vi "VGC Defaults.vi"() -> (3 "Data":T1={"UI References"={"Exit Ref"=refnum, "Save Ref"=refnum, "Export Ref"=refnum, "Acquire Ref"=refnum, "Configure Ref"=refnum, "Graph Ref"=refnum, "Analyze Ref"=refnum, "Status Ref"=refnum, "Snapshot Ref"=refnum, "Start Ref"=refnum}, "Vacuum Graph config"={"Log/Lin"=FALSE, "Show Backing"=FALSE, "Show Chamber"=FALSE}, "VGC50"={"serial settings"={"port"="Inficon_VGC503", "baud rate"=115200}, "device information"={"type"="", "model number"="", "serial number"="", "firmware version"="", "hardware version"=""}, "VGC"=refnum, "Backing SP"={"mode"=2, "thresholds"={"lower"=0.1, "upper"=1.0}, "on"=FALSE}, "Chamber SP"={"mode"=3, "thresholds"={"lower"=1e-05, "upper"=0.0001}, "on"=FALSE}}} {"VGC50"."Chamber SP"."thresholds"."upper" format="%#_5p"; "VGC50"."Chamber SP"."thresholds"."lower" format="%#_5p"; "VGC50"."Chamber SP"."mode" items=["off", "on", "channel 1", "channel 2", "channel 3"]; "VGC50"."Backing SP"."thresholds"."upper" format="%#_5p"; "VGC50"."Backing SP"."thresholds"."lower" format="%#_5p"; "VGC50"."Backing SP"."mode" items=["off", "on", "channel 1", "channel 2", "channel 3"]; "VGC50"."serial settings"."baud rate" items=["9600"=9600, "19200"=19200, "38400"=38400, "57600"=57600, "115200"=115200]})   [LabVIEW 2024]
uses:
  controls/UI References.ctl
  controls/Vac Graph Config.ctl
  Program Files/National Instruments/LabVIEW 2024/instr.lib/PL Inficon VGC/PL Inficon VGC.lvclass
  controls/VGC50.ctl
  controls/VGCData.ctl
panel:
  in  "VGC50":T4={"serial settings"={"port"="Inficon_VGC503", "baud rate"=115200}, "device information"={"type"="", "model number"="", "serial number"="", "firmware version"="", "hardware version"=""}, "VGC"=refnum, "Backing SP"={"mode"=2, "thresholds"={"lower"=0.0001, "upper"=0.005}, "on"=FALSE}, "Chamber SP"={"mode"=3, "thresholds"={"lower"=1e-05, "upper"=0.0001}, "on"=FALSE}} {"Chamber SP"."thresholds"."upper" format="%#_5p"; "Chamber SP"."thresholds"."lower" format="%#_5p"; "Chamber SP"."mode" items=["off", "on", "channel 1", "channel 2", "channel 3"]; "Backing SP"."thresholds"."upper" format="%#_5p"; "Backing SP"."thresholds"."lower" format="%#_5p"; "Backing SP"."mode" items=["off", "on", "channel 1", "channel 2", "channel 3"]; "serial settings"."baud rate" items=["9600"=9600, "19200"=19200, "38400"=38400, "57600"=57600, "115200"=115200]}
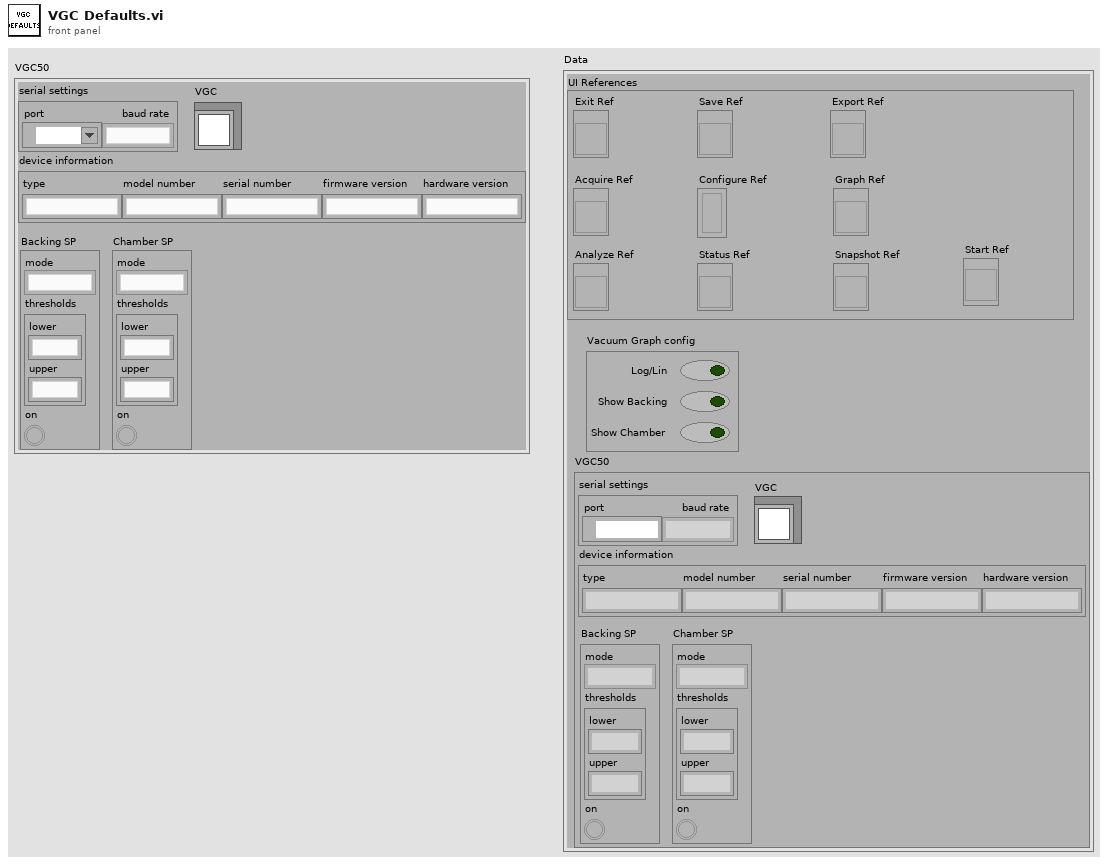
[diagram p1: front panel]
types:
  T1 = typedef "VGCData.ctl" = cluster{"UI References":T2, "Vacuum Graph config":T3, "VGC50":T4}
  T2 = typedef "UI References.ctl" = cluster{"Exit Ref":refnum<vi>, "Save Ref":refnum<vi>, "Export Ref":refnum<vi>, "Acquire Ref":refnum<vi>, "Configure Ref":refnum<vi>, "Graph Ref":refnum<vi>, "Analyze Ref":refnum<vi>, "Status Ref":refnum<vi>, "Snapshot Ref":refnum<vi>, "Start Ref":refnum<vi>}
  T3 = typedef "Vac Graph Config.ctl" = cluster{"Log/Lin":bool, "Show Backing":bool, "Show Chamber":bool}
  T4 = typedef "VGC50.ctl" = cluster{"serial settings":cluster{"port":refnum<visa-resource-name>, "baud rate":u32}, "device information":cluster{"type":string, "model number":string, "serial number":string, "firmware version":string, "hardware version":string}, "VGC":refnum<class "PL Inficon VGC.lvclass">, "Backing SP":cluster{"mode":u16, "thresholds":cluster{"lower":dbl, "upper":dbl}, "on":bool}, "Chamber SP":cluster{"mode":u16, "thresholds":cluster{"lower":dbl, "upper":dbl}, "on":bool}}
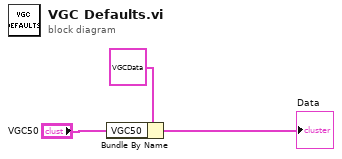
[diagram p0: block diagram]
diagram:
  n1 = Bundle By Name(cluster=T1 {"UI References"={"Exit Ref"=refnum, "Save Ref"=refnum, "Export Ref"=refnum, "Acquire Ref"=refnum, "Configure Ref"=refnum, "Graph Ref"=refnum, "Analyze Ref"=refnum, "Status Ref"=refnum, "Snapshot Ref"=refnum, "Start Ref"=refnum}, "Vacuum Graph config"={"Log/Lin"=FALSE, "Show Backing"=FALSE, "Show Chamber"=FALSE}, "VGC50"={"serial settings"={"port"="Inficon_VGC503", "baud rate"=115200}, "device information"={"type"="", "model number"="", "serial number"="", "firmware version"="", "hardware version"=""}, "VGC"=refnum, "Backing SP"={"mode"=2, "thresholds"={"lower"=0.1, "upper"=1.0}, "on"=FALSE}, "Chamber SP"={"mode"=3, "thresholds"={"lower"=1e-05, "upper"=0.0001}, "on"=FALSE}}} ("Data"), "VGC50"="VGC50") -> (→"Data":T1)
